vi "USB6343_Control_v1.3(1).vi"   [LabVIEW 2013]
uses:
  <vilib>/DAQmx/read.llb/DAQmx Read (Digital 1D Bool NChan 1Samp 1Line).vi
  <vilib>/DAQmx/read.llb/DAQmx Read (Analog 1D DBL NChan 1Samp).vi
  <vilib>/DAQmx/read.llb/DAQmx Read (Counter DBL 1Chan 1Samp).vi
  <vilib>/DAQmx/write.llb/DAQmx Write (Digital 1D Bool NChan 1Samp 1Line).vi
  <vilib>/DAQmx/write.llb/DAQmx Write (Analog 1D DBL NChan 1Samp).vi
  <vilib>/DAQmx/miscellaneous.llb/DAQmx Fill In Error Info.vi
types:
  T1 = cluster{"source":string, "channel":i32, "old value":dbl, "new value":dbl, "on/off":bool}
  T2 = cluster{"cmd":string, "channel":i32, "value":dbl, "on/off":bool, "return value":refnum<vi>}
  T3 = cluster{"AI Task":refnum<k21>, "AO Task":refnum<k21>, "DO Task":refnum<k21>, "DI Task":refnum<k21>}
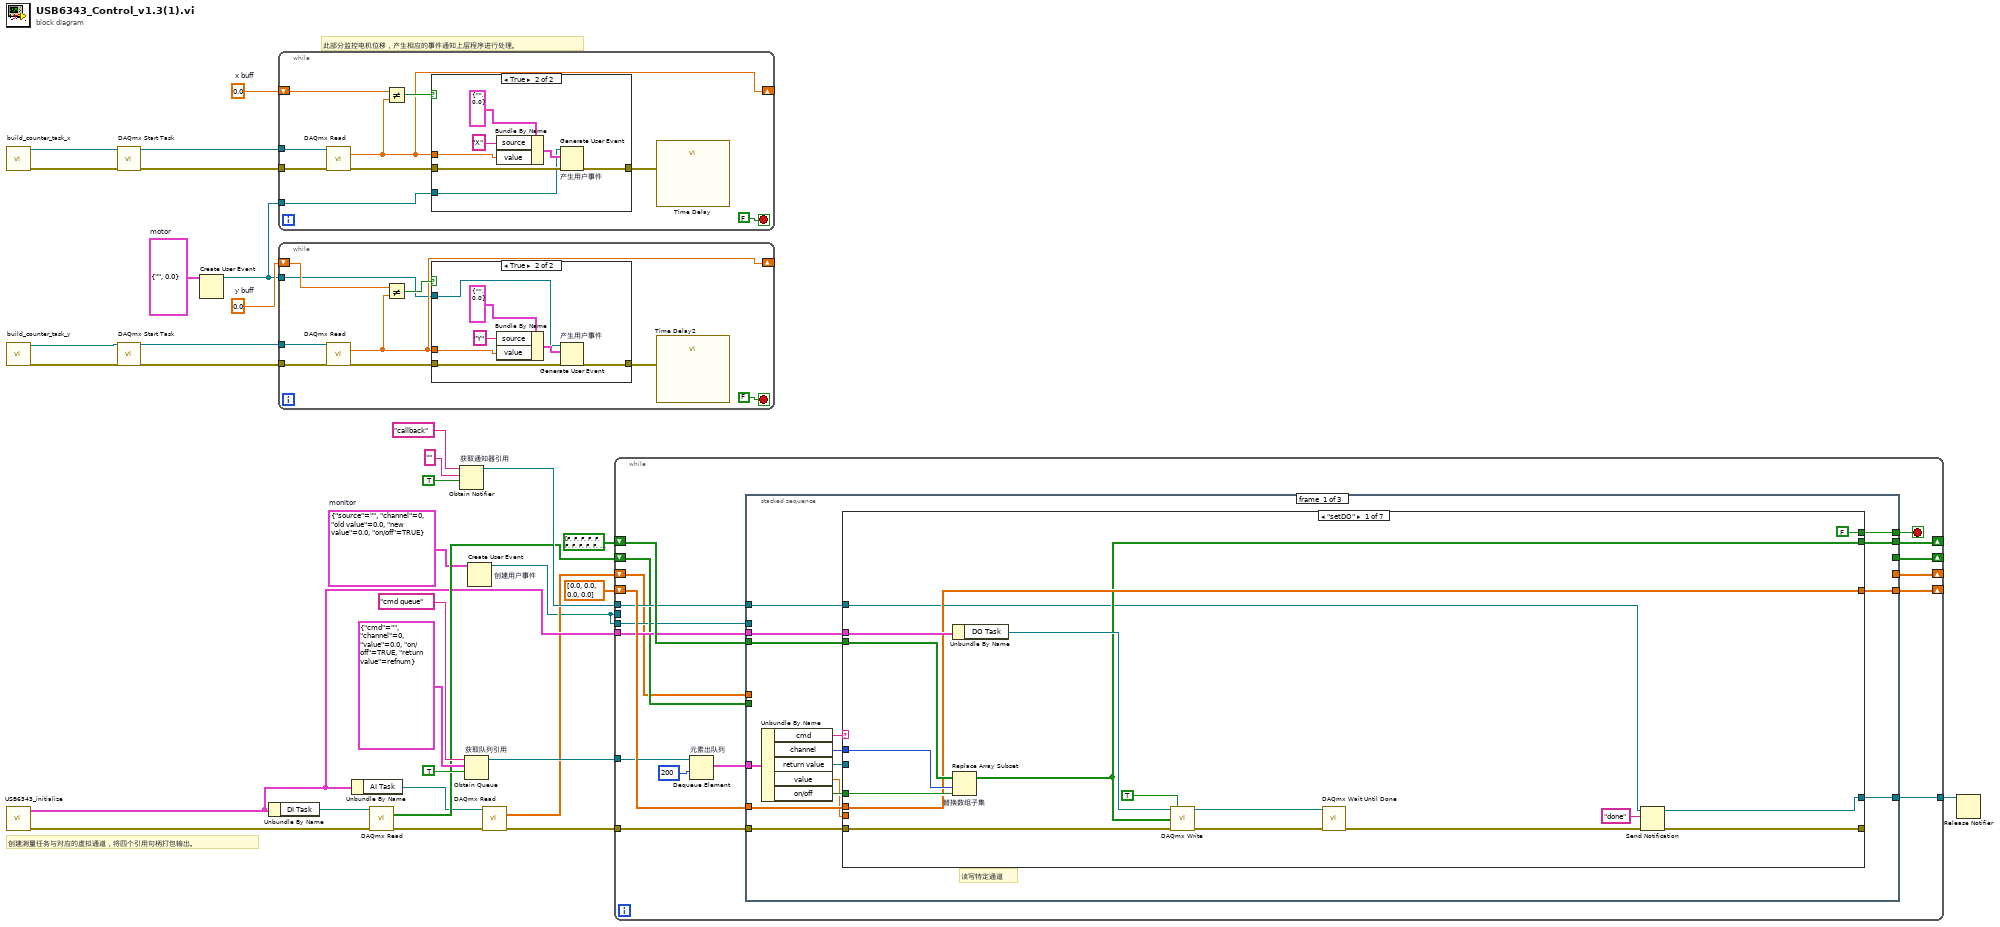
[diagram p0: block diagram]
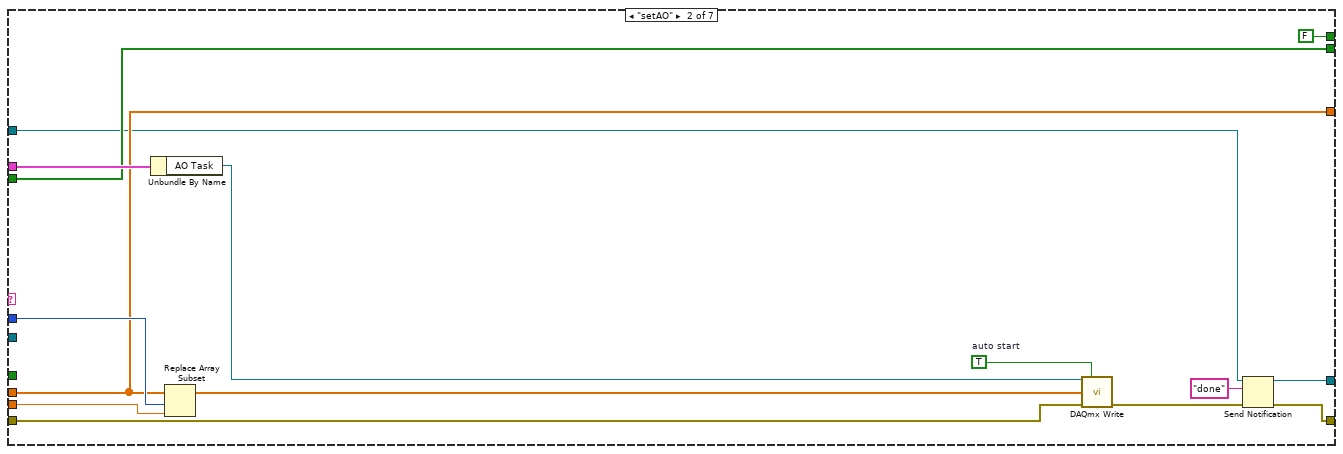
[diagram p4: hidden frame]
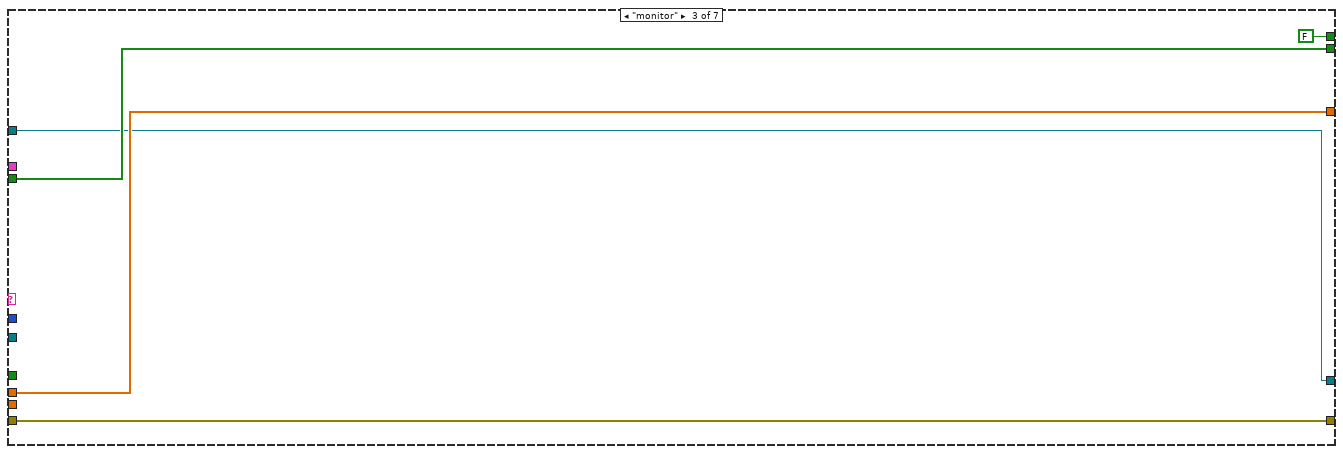
[diagram p5: hidden frame]
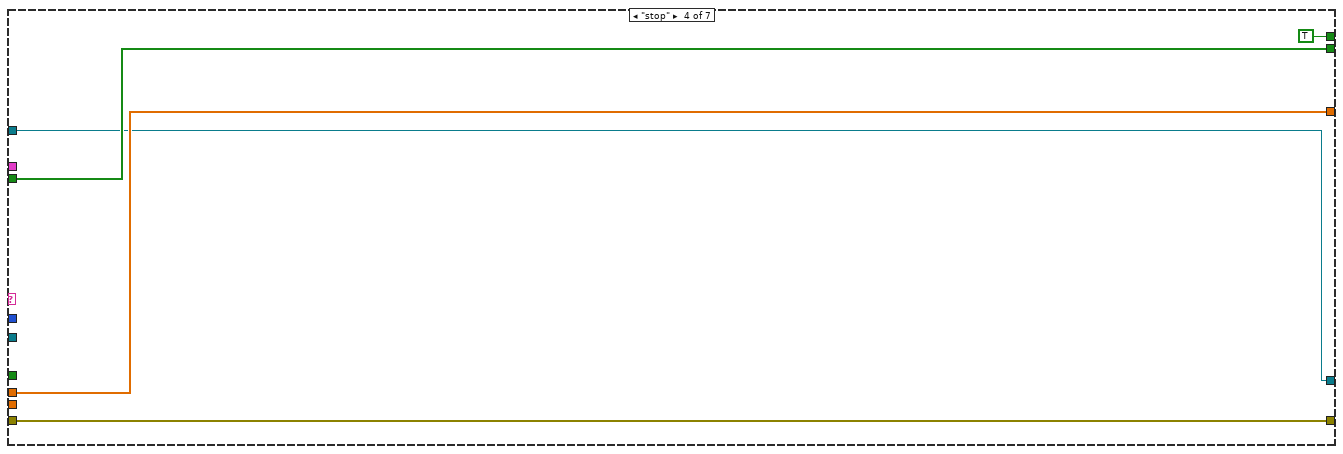
[diagram p6: hidden frame]
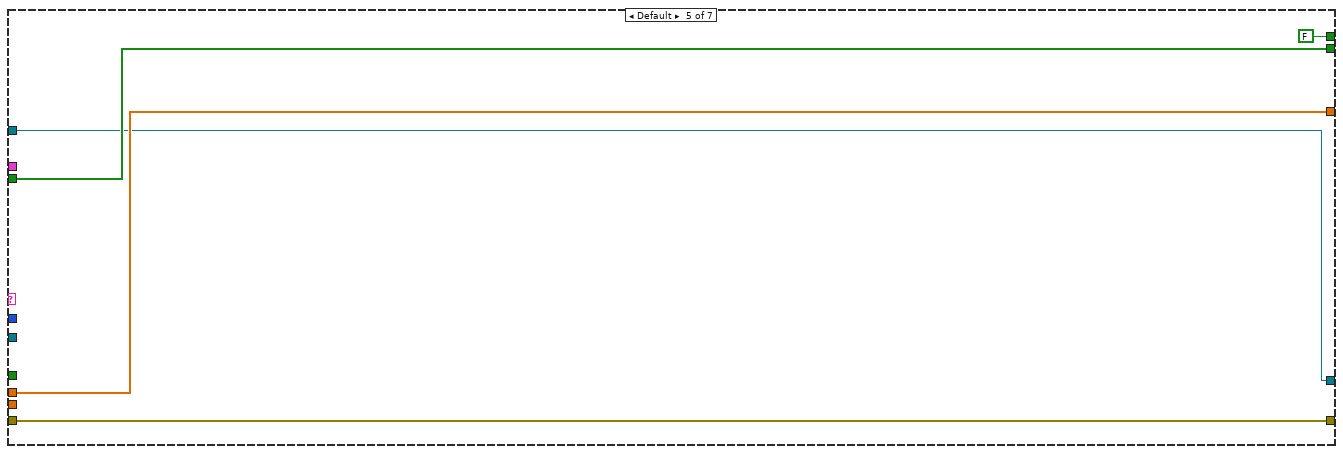
[diagram p7: hidden frame]
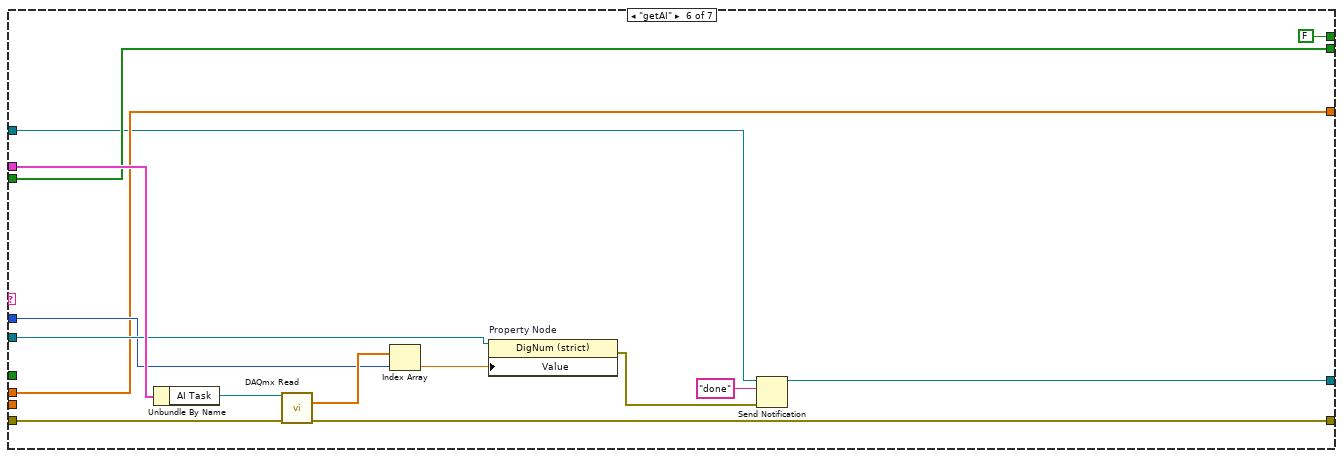
[diagram p8: hidden frame]
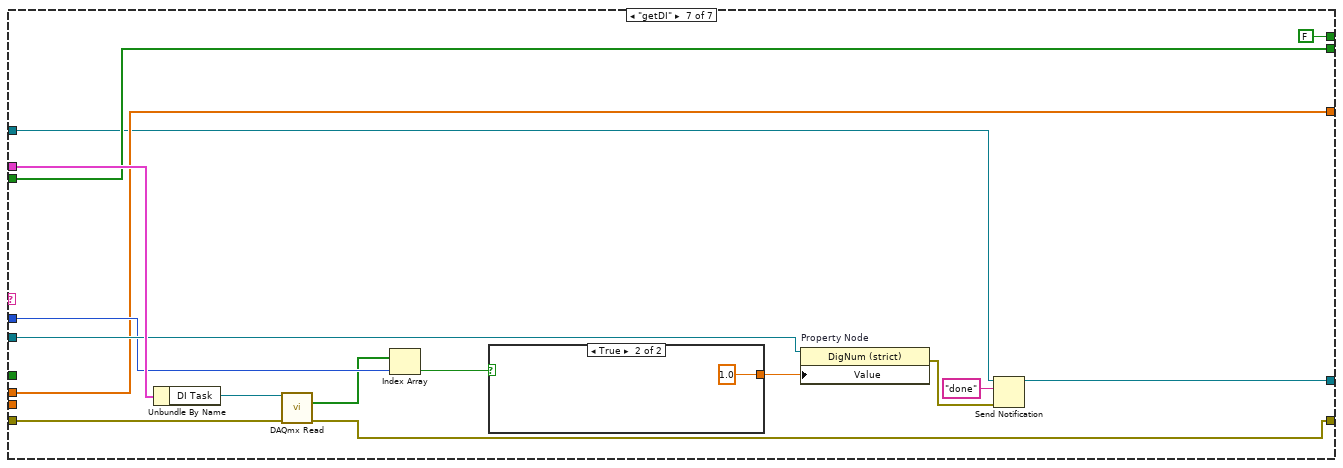
[diagram p9: hidden frame]
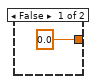
[diagram p10: hidden frame]
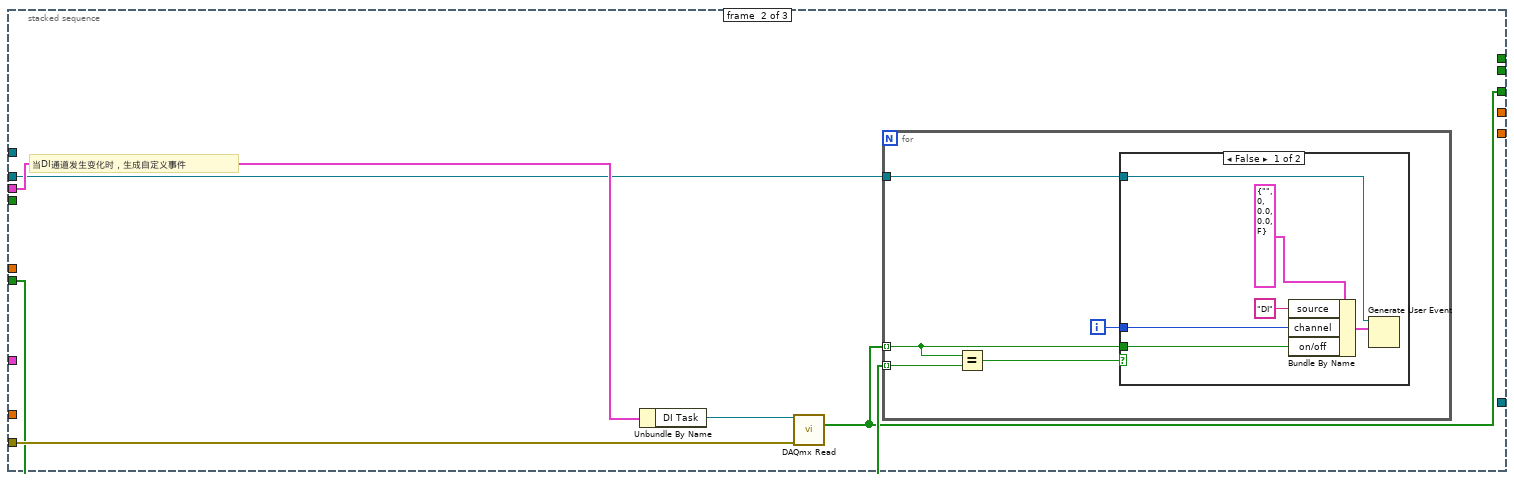
[diagram p11: hidden frame]
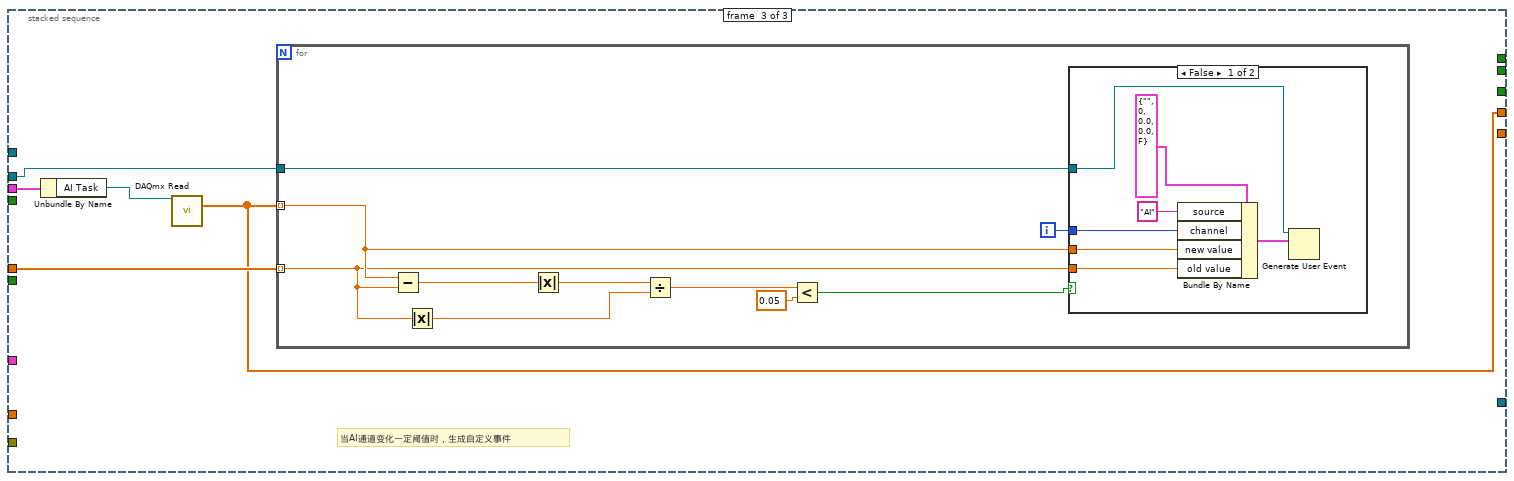
[diagram p13: hidden frame]
diagram:
  w2 = cluster{"source":string, "value":dbl} {"source"="", "value"=0.0}  # motor
  w4 = T1 {"source"="", "channel"=0, "old value"=0.0, "new value"=0.0, "on/off"=TRUE}  # monitor
  w26 = 0.0  # x buff
  w29 = 0.0  # y buff
  # "此部分监控电机位移，产生相应的事件通知上层程序进行处理。"
  # "创建测量任务与对应的虚拟通道，将四个引用句柄打包输出。"
  n1 = call "build_counter_task_x.vi"() -> ("error out"=w25:errorcluster, "task out"=w24:refnum<k21>)  [unwired: 10 in]
  n2 = call "build_counter_task_y.vi"() -> ("error out"=w22:errorcluster, "task out"=w23:refnum<k21>)  [unwired: 10 in]
  n3 = call "USB6343_initialize.vi"() -> ("error out"=w10:errorcluster, "tasks"=w7:T3)  [unwired: 10 in]
  n4 = call <vilib>:"DAQmx Start Task.vi"("task/channels in"=w24, "error in"=w25) -> ("task out"=w28:refnum<k21>, "error out"=w27:errorcluster)  [unwired: 12 in]
  n5 = call <vilib>:"DAQmx Start Task.vi"("task/channels in"=w23, "error in"=w22) -> ("task out"=w31:refnum<k21>, "error out"=w30:errorcluster)  [unwired: 12 in]
  n6 = Create User Event(user event datatype=w2) -> (user event=w1:refnum<user-event>)  [unwired: 1 in, 1 out]
  n7 = Unbundle By Name(w7) -> ("DI Task"=w12:refnum<k21>)
  n8 = while {
    tunnel: w28 -> [w40]
    tunnel: w27 -> [w42]
    shift-right: [w38] -> _
    shift-left: w26 -> [w41]
    tunnel: w1 -> [w34]
    stop <- FALSE stop-if-true
    n9 = call-poly <vilib>:"DAQmx Read.vi"("task/channels in"=w40, "error in"=w42) -> ("data"=w38:dbl, "error out"=w37:errorcluster)  [unwired: 11 in, 1 out]
    n10 = Not Equal?(x=w41, y=w38) -> (x != y?=w39:bool)
    n11 = case shown="True" w39 {
      tunnel: w38 -> [_ w48]
      tunnel: w37 -> [w43 w46]
      tunnel: [w43 w45] -> w35
      tunnel: w34 -> [_ w44]
      frame False {
      }
      frame True {
        n12 = Bundle By Name(cluster=cluster{"source":string, "value":dbl} {"source"="", "value"=0.0} ("事件数据"), "source"="X", "value"=w48) -> (w47:cluster{"source":string, "value":dbl})
        n13 = Generate User Event "产生用户事件"(user event=w44, event data cluster=w47, error in=w46) -> (error out=w45:errorcluster)  [unwired: 1 in, 1 out]
      }
    }
    n14 = call "Time Delay"("error in (no error)"=w35) -> ()  [unwired: 10 in, 1 out]
  }
  n15 = while {
    tunnel: w31 -> [w57]
    tunnel: w30 -> [w59]
    shift-right: [w55] -> _
    shift-left: w29 -> [w58]
    tunnel: w1 -> [w51]
    stop <- FALSE stop-if-true
    n16 = call-poly <vilib>:"DAQmx Read.vi"("task/channels in"=w57, "error in"=w59) -> ("data"=w55:dbl, "error out"=w54:errorcluster)  [unwired: 11 in, 1 out]
    n17 = Not Equal?(x=w58, y=w55) -> (x != y?=w56:bool)
    n18 = case shown="True" w56 {
      tunnel: w55 -> [_ w61]
      tunnel: w54 -> [w60 w63]
      tunnel: [w60 w62] -> w52
      tunnel: w51 -> [_ w64]
      frame False {
      }
      frame True {
        n19 = Bundle By Name(cluster=cluster{"source":string, "value":dbl} {"source"="", "value"=0.0} ("事件数据"), "source"="Y", "value"=w61) -> (w65:cluster{"source":string, "value":dbl})
        n20 = Generate User Event "产生用户事件"(user event=w64, event data cluster=w65, error in=w63) -> (error out=w62:errorcluster)  [unwired: 1 in, 1 out]
      }
    }
    n21 = call "Time Delay2"("error in (no error)"=w52) -> ()  [unwired: 10 in, 1 out]
  }
  n22 = Unbundle By Name(w7) -> ("AI Task"=w6:refnum<k21>)
  n23 = call-poly <vilib>:"DAQmx Read.vi"("task/channels in"=w12, "error in"=w10) -> ("data"=w11:bool[], "error out"=w9:errorcluster)  [unwired: 11 in, 1 out]
  n24 = Obtain Notifier "获取通知器引用"(name (unnamed)="callback" ("名称（未命名）"), notification data type="", create if not found? (T)=TRUE ("如未找到是否创建？(T)")) -> (notifier out=w15:refnum<notifier>)  [unwired: 1 in, 2 out]
  n25 = Obtain Queue "获取队列引用"(name (unnamed)="cmd queue" ("名称（未命名）"), element data type=T2 {"cmd"="", "channel"=0, "value"=0.0, "on/off"=TRUE, "return value"=refnum}, create if not found? (T)=TRUE ("如未找到是否创建？(T)")) -> (queue out=w19:refnum<queue>)  [unwired: 2 in, 2 out]
  n26 = Create User Event "创建用户事件"(user event datatype=w4) -> (user event=w3:refnum<user-event>)  [unwired: 1 in, 1 out]
  n27 = call-poly <vilib>:"DAQmx Read.vi"("task/channels in"=w6, "error in"=w9) -> ("data"=w5:dbl[], "error out"=w8:errorcluster)  [unwired: 11 in, 1 out]
  n28 = while {
    tunnel: w7 -> [w78]
    tunnel: w8 -> [w84]
    shift-right: [w82] -> _
    shift-left: bool[] [FALSE, FALSE, FALSE, FALSE, FALSE, FALSE, FALSE, FALSE, FALSE, FALSE, FALSE, FALSE, FALSE, FALSE, FALSE, FALSE] -> [w83]
    shift-right: [w79] -> _
    shift-left: dbl[] [0.0, 0.0, 0.0, 0.0] ("data") -> [w80]
    tunnel: w19 -> [w77]
    tunnel: w15 -> [w74]
    tunnel: [w73] -> w14
    shift-right: [w71] -> _
    shift-left: w11 -> [w72]
    shift-right: [w68] -> _
    shift-left: w5 -> [w69]
    tunnel: w3 -> [w70]
    tunnel: w3 -> [_]
    stop <- w81 stop-if-true
    n29 = Dequeue Element "元素出队列"(queue=w77, timeout in ms (-1)=200 ("超时毫秒(-1)")) -> (element=w76:T2)  [unwired: 1 in, 3 out]
    n30 = stacked-sequence {
      tunnel: w84 -> [w99 w183 _]
      tunnel: w83 -> [w98 _ _]
      tunnel: [w97 _ _] -> w82
      tunnel: [w96 _ _] -> w81
      tunnel: w80 -> [w95 _ _]
      tunnel: [w94 _ _] -> w79
      tunnel: w78 -> [w85 w185 w201]
      tunnel: w76 -> [w93 _ _]
      tunnel: w74 -> [w87 _ _]
      tunnel: [w86 _ _] -> w73
      tunnel: w72 -> [_ w182 _]
      tunnel: [_ w181 _] -> w71
      tunnel: w70 -> [_ w180 w197]
      tunnel: w69 -> [_ _ w199]
      tunnel: [_ _ w198] -> w68
      frame #0 {
        # "读写特定通道"
        n31 = Unbundle By Name(w93) -> ("cmd"=w92:string, "channel"=w91:i32, "return value"=w90:refnum<vi>, "value"=w88:dbl, "on/off"=w89:bool)
        n32 = case shown="\"setDO\"" w92 {
          tunnel: w91 -> [w114 w129 _ _ _ w156 w175]
          tunnel: w85 -> [w116 w131 _ _ _ w161 w177]
          tunnel: w99 -> [w108 w123 w133 w138 w143 w158 w167]
          tunnel: w98 -> [w115 w127 w136 w141 w146 w154 w174]
          tunnel: w89 -> [w113 _ _ _ _ _ _]
          tunnel: [w106 w127 w136 w141 w146 w154 w174] -> w97
          tunnel: [FALSE FALSE FALSE TRUE FALSE FALSE FALSE] -> w96
          tunnel: w95 -> [w111 w128 w135 w139 w144 w153 w173]
          tunnel: [w111 w128 w135 w139 w144 w153 w173] -> w94
          tunnel: w90 -> [_ _ _ _ _ w159 w176]
          tunnel: [w110 w121 w133 w138 w143 w151 w166] -> _
          tunnel: w88 -> [_ w119 _ _ _ _ _]
          tunnel: w87 -> [w101 w118 w132 w137 w142 w148 w169]
          tunnel: [w100 w117 w132 w137 w142 w147 w168] -> w86
          frame "setDO" {
            n33 = Unbundle By Name(w116) -> ("DO Task"=w107:refnum<k21>)
            n34 = Replace Array Subset "替换数组子集"(array=w115, new element=w113, index=w114) -> (w106:bool[])
            n35 = call-poly <vilib>:"DAQmx Write.vi"("task/channels in"=w107, "auto start"=TRUE, "data"=w106, "error in"=w108) -> ("task out"=w102:refnum<k21>, "error out"=w104:errorcluster)  [unwired: 9 in, 1 out]
            n36 = call <vilib>:"DAQmx Wait Until Done.vi"("task/channels in"=w102, "error in"=w104) -> ("error out"=w103:errorcluster)  [unwired: 12 in, 1 out]
            n37 = Send Notification(notification="done" ("通知"), notifier=w101, error in (no error)=w103) -> (notifier out=w100:refnum<notifier>, error out=w110:errorcluster)
          }
          frame "setAO" {
            w125 = TRUE  # auto start
            n38 = Unbundle By Name(w131) -> ("AO Task"=w130:refnum<k21>)
            n39 = Replace Array Subset(array=w128, new element=w119, index=w129) -> (w126:dbl[])
            n40 = call-poly <vilib>:"DAQmx Write.vi"("task/channels in"=w130, "auto start"=w125, "data"=w126, "error in"=w123) -> ("error out"=w122:errorcluster)  [unwired: 9 in, 2 out]
            n41 = Send Notification(notification="done" ("通知"), notifier=w118, error in (no error)=w122) -> (notifier out=w117:refnum<notifier>, error out=w121:errorcluster)
          }
          frame "monitor" {
          }
          frame "stop" {
          }
          frame Default {
          }
          frame "getAI" {
            n42 = Unbundle By Name(w161) -> ("AI Task"=w160:refnum<k21>)
            n43 = call-poly <vilib>:"DAQmx Read.vi"("task/channels in"=w160, "error in"=w158) -> ("data"=w157:dbl[], "error out"=w151:errorcluster)  [unwired: 11 in, 1 out]
            n44 = Index Array(array=w157, index=w156) -> (element=w155:dbl)
            n45 = property on="Property Node" class="DigNum (strict)"(reference=w159, "Value"=w155) -> (error out=w149:errorcluster)  [unwired: 1 in, 1 out]
            n46 = Send Notification(notification="done" ("通知"), notifier=w148, error in (no error)=w149) -> (notifier out=w147:refnum<notifier>)  [unwired: 1 out]
          }
          frame "getDI" {
            n47 = Unbundle By Name(w177) -> ("DI Task"=w165:refnum<k21>)
            n48 = call-poly <vilib>:"DAQmx Read.vi"("task/channels in"=w165, "error in"=w167) -> ("data"=w164:bool[], "error out"=w166:errorcluster)  [unwired: 11 in, 1 out]
            n49 = Index Array(array=w164, index=w175) -> (element=w163:bool)
            n50 = case shown="True" w163 {
              tunnel: [0.0 1.0] -> w162
              frame False {
              }
              frame True {
              }
            }
            n51 = property on="Property Node" class="DigNum (strict)"(reference=w176, "Value"=w162) -> (error out=w170:errorcluster)  [unwired: 1 in, 1 out]
            n52 = Send Notification(notification="done" ("通知"), notifier=w169, error in (no error)=w170) -> (notifier out=w168:refnum<notifier>)  [unwired: 1 out]
          }
        }
      }
      frame #1 {
        # "当DI通道发生变化时，生成自定义事件"
        n53 = Unbundle By Name(w185) -> ("DI Task"=w184:refnum<k21>)
        n54 = call-poly <vilib>:"DAQmx Read.vi"("task/channels in"=w184, "error in"=w183) -> ("data"=w181:bool[])  [unwired: 11 in, 2 out]
        n55 = for {
          tunnel: w181 -> [w186] mode=indexing
          tunnel: w182 -> [w190] mode=indexing
          tunnel: w180 -> [w187]
          i -> [w188]
          n56 = Equal?(x=w186, y=w190) -> (x = y?=w189:bool)
          n57 = case shown="False" w189 {
            tunnel: w188 -> [w193 _]
            tunnel: w187 -> [w196 _]
            tunnel: w186 -> [w192 _]
            frame False {
              n58 = Bundle By Name(cluster=T1 {"source"="", "channel"=0, "old value"=0.0, "new value"=0.0, "on/off"=FALSE} ("事件数据"), "source"="DI", "channel"=w193, "on/off"=w192) -> (w191:T1)
              n59 = Generate User Event(user event=w196, event data cluster=w191) -> ()  [unwired: 2 in, 2 out]
            }
            frame True {
            }
          }
        }
      }
      frame #2 {
        # "当AI通道变化一定阈值时，生成自定义事件"
        n60 = Unbundle By Name(w201) -> ("AI Task"=w200:refnum<k21>)
        n61 = call-poly <vilib>:"DAQmx Read.vi"("task/channels in"=w200) -> ("data"=w198:dbl[])  [unwired: 12 in, 2 out]
        n62 = for {
          tunnel: w198 -> [w203] mode=indexing
          tunnel: w199 -> [w202] mode=indexing
          tunnel: w197 -> [w205]
          i -> [w204]
          n63 = Subtract(x=w203, y=w202) -> (x-y=w211:dbl)
          n64 = Absolute Value(x=w202) -> (abs(x)=w209:dbl)
          n65 = Absolute Value(x=w211) -> (abs(x)=w210:dbl)
          n66 = Divide(x=w210, y=w209) -> (x/y=w208:dbl)
          n67 = Less?(x=w208, y=0.05) -> (x < y?=w206:bool)
          n68 = case shown="False" w206 {
            tunnel: w205 -> [w218 _]
            tunnel: w204 -> [w215 _]
            tunnel: w203 -> [w214 _]
            tunnel: w202 -> [w213 _]
            frame False {
              n69 = Bundle By Name(cluster=T1 {"source"="", "channel"=0, "old value"=0.0, "new value"=0.0, "on/off"=FALSE} ("事件数据"), "source"="AI", "channel"=w215, "new value"=w214, "old value"=w213) -> (w212:T1)
              n70 = Generate User Event(user event=w218, event data cluster=w212) -> ()  [unwired: 2 in, 2 out]
            }
            frame True {
            }
          }
        }
      }
    }
  }
  n71 = Release Notifier(notifier=w14) -> ()  [unwired: 2 in, 3 out]
